vi "OpenCV Canny Function.vi"() -> ()   [LabVIEW 2017]
uses:
  IMAQCV/IMAQCV.lvlib
  IMAQCV/LVOpenCV.lvlib
  IMAQCV/PIIO.lvlib
panel:
  out "Loop Rate (Hz)":u32
  in  "Image Size":T1(ring)
  out "error out":errorcluster
  in  "Canny Options":T2={"threshold1"=250, "threshold2"=90, "apertureSize"=3, "L2gradient"=0} {"apertureSize" items=["3"=3, "5"=5, "7"=7]}
  out "count":i32
  out "Output":picture caption="Output 2"
  out "Input":picture caption="Output"
  in  "stop":bool
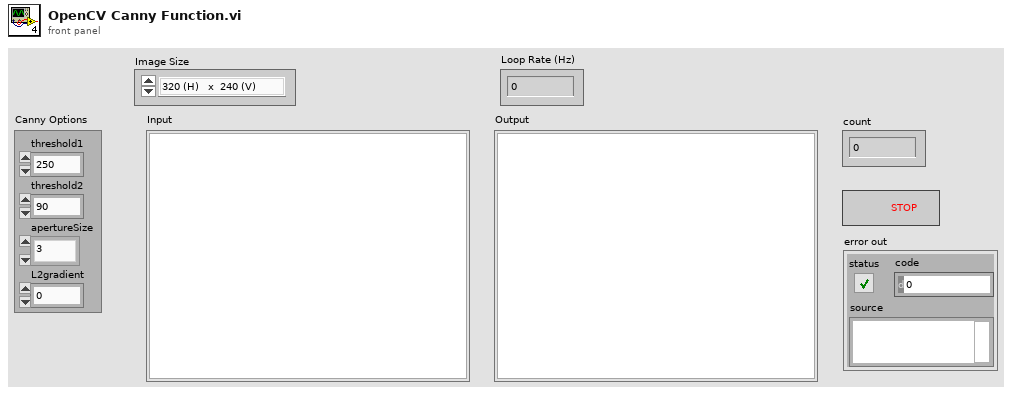
[diagram p1: front panel]
types:
  T1 = enum16{"320 (H)   x  240 (V)", "352(H)    x  288 (V)", "640 (H)   x  480 (V) ", "800 (H)   x  600 (V)", "1024 (H) x  768 (V)", "1280 (H) x  720 (V)", "1280 (H) x  960 (V)", "1280 (H) x 1024 (V)", "1920 (H) x 1080 (V)"}
  T2 = cluster{"threshold1":i32, "threshold2":i32, "apertureSize":i32, "L2gradient":i8}
  T3 = typedef "IMAQCV.lvlib/IMAQCV Image.ctl" = refnum<vi>
  T4 = typedef "Image Type" = u32
  T5 = cluster{"Image Type":T4, "height":i32, "width":i32, "depth":i32, "channels":i32}
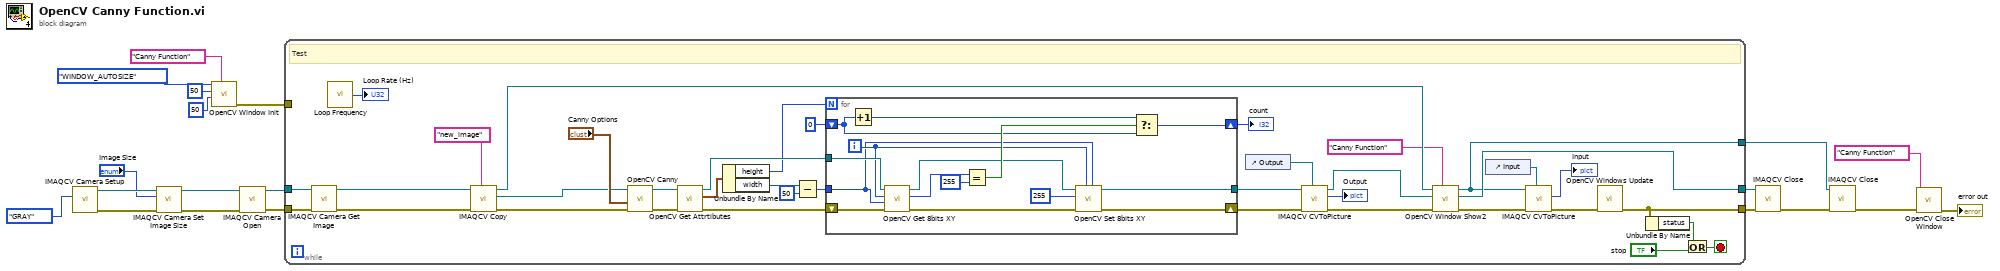
[diagram p0: block diagram]
diagram:
  n1 = call "IMAQCV Camera Setup.vi"("type"=enum16{"GRAY", "COLOR"}."GRAY") -> ("error out"=w6:errorcluster, "image out"=w4:T3)  [unwired: 9 in]
  n2 = call "IMAQCV Camera Set Image Size.vi"("error in (no error)"=w6, "Image Size"="Image Size", "image in"=w4) -> ("error out"=w7:errorcluster, "image out"=w3:T3)  [unwired: 7 in]
  n3 = call "OpenCV Window Init.vi"("window name"="Canny Function", "y"=u32 50, "x"=u32 50, "mode"=enum8{"WINDOW_AUTOSIZE", "WINDOW_FULLSCREEN"}."WINDOW_AUTOSIZE") -> ("error out"=w9:errorcluster)  [unwired: 7 in]
  n4 = call "IMAQCV Camera Open.vi"("error in (no error)"=w7, "image in"=w3) -> ("error out"=w8:errorcluster, "image out"=w2:T3)  [unwired: 8 in]
  n5 = while {
    tunnel: w8 -> [w52]
    tunnel: [w32] -> w19
    tunnel: w2 -> [w51]
    tunnel: [w41] -> w20
    tunnel: [w40] -> w17
    tunnel: w9 -> [_]
    stop <- w34 stop-if-true
    # "Test"
    n6 = call "IMAQCV Camera Get Image.vi"("error in (no error)"=w52, "image in"=w51) -> ("error out"=w29:errorcluster, "image out"=w28:T3)  [unwired: 8 in]
    n7 = call "Loop Frequency.vi"() -> ("Loop Rate (Hz)"=→"Loop Rate (Hz)":u32)  [unwired: 1 out]
    n8 = call "IMAQCV Copy.vi"("New Image Name"="new_image", "error in (no error)"=w29, "Image Src"=w28) -> ("error out"=w27:errorcluster, "Image Dst Out"=w26:T3, "Image Src Out"=w38:T3)  [unwired: 5 in]
    n9 = call "OpenCV Canny.vi"("error in (no error)"=w27, "Canny Options"="Canny Options", "image"=w26) -> ("error out"=w49:errorcluster, "image out"=w47:T3)  [unwired: 7 in]
    n10 = call "OpenCV Get Attrtibutes.vi"("error in (no error)"=w49, "edges in"=w47) -> ("error out"=w45:errorcluster, "attr"=w50:T5, "image out"=w48:T3)  [unwired: 7 in]
    n11 = Unbundle By Name(w50) -> ("height"=w46:i32, "width"=w44:i32)
    n12 = Subtract(x=w44, y=50) -> (x-y=w57:i32)
    n13 = for {
      N: w46 -> [_]
      tunnel: w48 -> [w62]
      tunnel: w57 -> [w59]
      shift-right: [w68] -> w55
      shift-left: 0 -> [w69]
      tunnel: [w64] -> w37
      shift-right: [w65] -> w36
      shift-left: w45 -> [w67]
      i -> [w60]
      n14 = Increment(x=w69) -> (x+1=w70:i32)
      n15 = call "OpenCV Get 8bits XY.vi"("error in (no error)"=w67, "y"=w59, "x"=w60, "image in"=w62) -> ("error out"=w66:errorcluster, "data"=w73:i32, "image out"=w63:T3)  [unwired: 5 in]
      n16 = Equal?(x=w73, y=255) -> (x = y?=w71:bool)
      n17 = call "OpenCV Set 8bits XY.vi"("y"=w59, "x"=w60, "error in (no error)"=w66, "data"=u8 255, "image in"=w63) -> ("error out"=w65:errorcluster, "image out"=w64:T3)  [unwired: 5 in]
      n18 = Select(t=w70, s=w71, f=w69) -> (s? t:f=w68:i32)
    }
    "count" <- w55
    n19 = control-ref of="Output"() -> (w22:refnum<vi>)
    n20 = call "IMAQCV CVToPicture.vi"("picture ref"=w22, "error in (no error)"=w36, "image"=w37) -> ("error out"=w24:errorcluster, "picture"=→"Output":picture, "image out"=w25:T3)  [unwired: 6 in]
    n21 = call "OpenCV Window Show2.vi"("title"="Canny Function", "error in (no error)"=w24, "image2"=w25, "image1"=w38) -> ("error out"=w39:errorcluster, "image2 out"=w41:T3, "image1 out"=w40:T3)  [unwired: 5 in]
    n22 = control-ref of="Input"() -> (w23:refnum<vi>)
    n23 = call "IMAQCV CVToPicture.vi"("picture ref"=w23, "error in (no error)"=w39, "image"=w40) -> ("error out"=w35:errorcluster, "picture"=→"Input":picture)  [unwired: 6 in, 1 out]
    n24 = call "OpenCV Windows Update.vi"("error in (no error)"=w35) -> ("error out"=w32:errorcluster)  [unwired: 9 in, 1 out]
    n25 = Unbundle By Name(w32) -> ("status"=w31:bool)
    n26 = Or(x=w31, y="stop") -> (x .or. y?=w34:bool)
  }
  n27 = call "IMAQCV Close.vi"("error in (no error)"=w19, "Image"=w20) -> ("error out"=w18:errorcluster)  [unwired: 9 in]
  n28 = call "IMAQCV Close.vi"("error in (no error)"=w18, "Image"=w17) -> ("error out"=w13:errorcluster)  [unwired: 9 in]
  n29 = call "OpenCV Close Window.vi"("error in (no error)"=w13, "window name"="Canny Function") -> ("error out"=→"error out":errorcluster)  [unwired: 9 in]
